vi "Create Tx IPv4 Frame.vi"(0 "Destination IP":u8[](array[numeric]), 1 "Frame ID":u8, 5 "Destination port":u16, 7 "RF data":string, 9 "Source port":u16, 11 "Protocol":T3, 12 "Transmit options bitfield":bool) -> (8 "TX IPv4 Frame":T1 {"Checksum" format="%x"; "Frame Type" items=["Frame Error"=254, "Device Response Status"=186, "Device Request"=185, "Send Data Response"=184, "RX Packet IPv4"=176, "Zigbee Remote AT Command Response"=151, "Explicit Zigbee Receive Packet"=145, "Zigbee Receive Packet"=144, "I/O Sample Rx Indicator"=143, "Zigbee TX Status"=139, "Modem Status"=138, "Transmit Status"=137, "AT Command Response"=136, "Remote Command Response"=135, "Rx Packet"=128, "Device Response"=42, "Send Data Request"=40, "TX Request IPv4"=32, "Zigbee Remote AT Command"=23, "Zigbee Explicit Transmit Packet"=17, "Zigbee Transmit Packet"=16, "AT Command "=8, "Remote AT Command Request"=7, "TX Request"=0]})   [LabVIEW 2016]
uses:
  WiFi API Frame Type.ctl
  WiFi API Frame.ctl
  Protocol enum.ctl
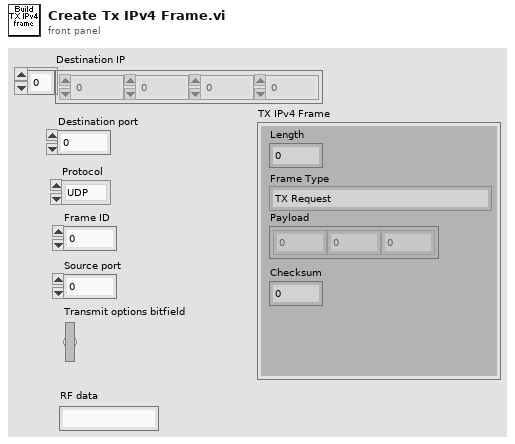
[diagram p1: front panel]
types:
  T1 = typedef "WiFi API Frame.ctl" = cluster{"Length":u16, "Frame Type":T2, "Payload":u8[], "Checksum":u8}
  T2 = typedef "WiFi API Frame Type.ctl" = u8
  T3 = typedef "Protocol enum.ctl" = enum8{"UDP", "TCP"}
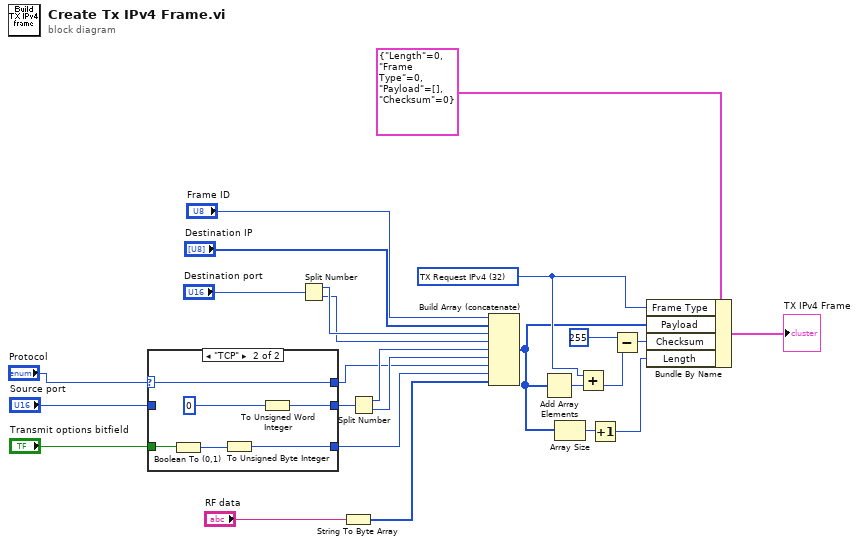
[diagram p0: block diagram]
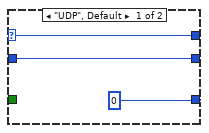
[diagram p2: hidden frame]
diagram:
  w5 = T2 32 items=["Frame Error"=254, "Device Response Status"=186, "Device Request"=185, "Send Data Response"=184, "RX Packet IPv4"=176, "Zigbee Remote AT Command Response"=151, "Explicit Zigbee Receive Packet"=145, "Zigbee Receive Packet"=144, "I/O Sample Rx Indicator"=143, "Zigbee TX Status"=139, "Modem Status"=138, "Transmit Status"=137, "AT Command Response"=136, "Remote Command Response"=135, "Rx Packet"=128, "Device Response"=42, "Send Data Request"=40, "TX Request IPv4"=32, "Zigbee Remote AT Command"=23, "Zigbee Explicit Transmit Packet"=17, "Zigbee Transmit Packet"=16, "AT Command "=8, "Remote AT Command Request"=7, "TX Request"=0] ("Frame Type")
  n1 = case shown="\"TCP\"" "Protocol" {
    selector: "Protocol" -> [w28 w30]
    tunnel: "Source port" -> [w27 _]
    tunnel: [w27 w29] -> w16
    tunnel: "Transmit options bitfield" -> [_ w33]
    tunnel: [u8 0 w31] -> w12
    tunnel: [w28 w30] -> w13
    frame "UDP", Default {
    }
    frame "TCP" {
      n2 = Boolean To (0,1)(Boolean=w33) -> (0, 1=w32:i16)
      n3 = To Unsigned Byte Integer(number=w32) -> (unsigned 8bit integer=w31:u8)
      n4 = To Unsigned Word Integer(number=u8 0) -> (unsigned 16bit integer=w29:u16)
    }
  }
  n5 = Split Number(x="Destination port") -> (hi(x)=w18:u8, lo(x)=w17:u8)
  n6 = String To Byte Array(string="RF data") -> (unsigned byte array=w10:u8[])
  n7 = Split Number(x=w16) -> (hi(x)=w15:u8, lo(x)=w14:u8)
  n8 = Build Array (concatenate)("Frame ID", "Destination IP", w18, w17, w15, w14, w13, w12, w10) -> (w4:u8[])
  n9 = Add Array Elements(numeric array=w4) -> (sum=w9:u8)
  n10 = Array Size(array=w4) -> (size(s)=w3:i32)
  n11 = Add(x=w5, y=w9) -> (x+y=w6:T2)
  n12 = Increment(x=w3) -> (x+1=w2:i32)
  n13 = Subtract(x=u8 255, y=w6) -> (x-y=w7:T2)
  n14 = Bundle By Name(cluster=T1 {"Length"=0, "Frame Type"=0, "Payload"=[], "Checksum"=0} ("API Frame"), "Frame Type"=w5, "Payload"=w4, "Checksum"=w7, "Length"=w2) -> (→"TX IPv4 Frame":T1)
